vi "tsdiag_can_routine_control.vi"(6 "ATimeoutMS":i32, 7 "ARoutintID":u16, 8 "错误输入（无错误）":errorcluster, 9 "ARoutineControlType":u8, 10 "ADiagModuleIndex":i32, 11 "path":path) -> (0 "错误输出":errorcluster, 2 "Return Type":i32, 3 "path out":path)   [LabVIEW 2014]
doc: "Function Introduction :\nSet CAN general control type value\nCall location :\ninput parameter :\nADiagModulus Index: Handle to UDS module\nARoutineControlType: Routine Control Type\nARoututID: Routine ID\nReturn value :\n==0: Execution successful\nOther values: Query error code"
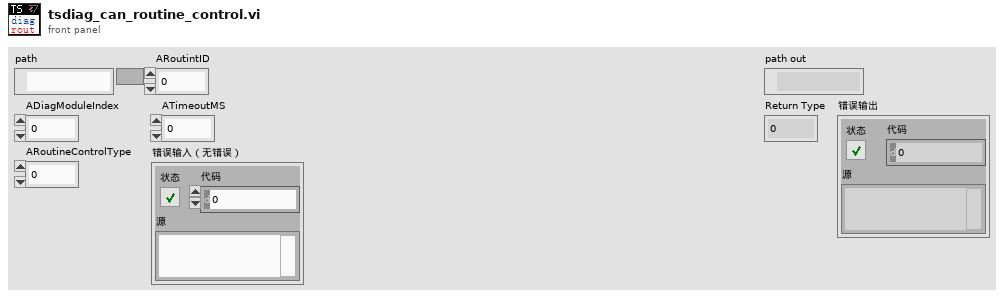
[diagram p1: front panel]
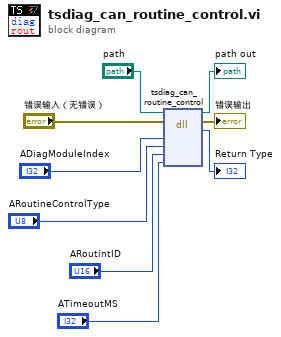
[diagram p0: block diagram]
diagram:
  n1 = dll-call lib="C:/Users/XYY/Desktop/LabView Demo/TSCAN_LB2018_V1.4_20220309/Config/TSMaster.dll" fn="tsdiag_can_routine_control"(path in="path", error in="错误输入（无错误）", "ADiagModuleIndex"="ADiagModuleIndex", "ARoutineControlType"="ARoutineControlType", "ARoutintID"="ARoutintID", "ATimeoutMS"="ATimeoutMS") -> (path out=→"path out":path, error out=→"错误输出":errorcluster, "返回类型"=→"Return Type":i32)  [unwired: 5 in]
